vi "ClimbDashReadNetwork.vi"() -> (0 "ReachLimit":bool, 1 "PullLimit":bool, 2 "SensorPosition":dbl, 3 "ClimbMotorDmd":dbl, 4 "ClimbStatus":string)   [LabVIEW 2023]
uses:
  <vilib>/Rock Robotics/Network Tables/NT Read Boolean.vi
  <vilib>/Rock Robotics/Network Tables/NT Read Number.vi
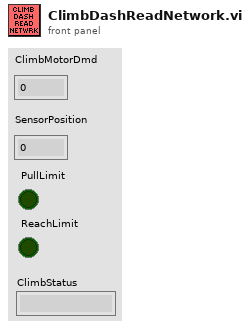
[diagram p1: front panel]
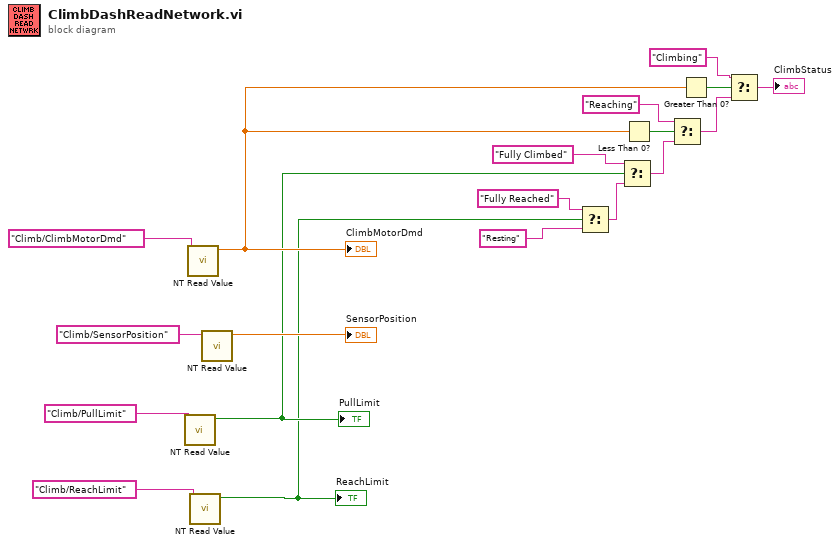
[diagram p0: block diagram]
diagram:
  n1 = call-poly <vilib>:"NT Read Value.vi"("name"="Climb/PullLimit") -> ("value"=w8:bool)  [unwired: 8 in, 2 out]
  "PullLimit" <- w8
  n2 = call-poly <vilib>:"NT Read Value.vi"("name"="Climb/ClimbMotorDmd") -> ("value"=w10:dbl)  [unwired: 8 in, 2 out]
  "ClimbMotorDmd" <- w10
  n3 = call-poly <vilib>:"NT Read Value.vi"("name"="Climb/ReachLimit") -> ("value"=w7:bool)  [unwired: 8 in, 2 out]
  "ReachLimit" <- w7
  n4 = call-poly <vilib>:"NT Read Value.vi"("name"="Climb/SensorPosition") -> ("value"=→"SensorPosition":dbl)  [unwired: 8 in, 2 out]
  n5 = Select(t="Fully Reached", s=w7, f="Resting") -> (s? t:f=w4:string)
  n6 = Select(t="Fully Climbed", s=w8, f=w4) -> (s? t:f=w5:string)
  n7 = Less Than 0?(x=w10) -> (x < 0?=w12:bool)
  n8 = Select(t="Reaching", s=w12, f=w5) -> (s? t:f=w9:string)
  n9 = Greater Than 0?(x=w10) -> (x > 0?=w14:bool)
  n10 = Select(t="Climbing", s=w14, f=w9) -> (s? t:f=→"ClimbStatus":string)
